vi "Datadashboard CD Main Page.vi"(8 "error in (no error)":errorcluster, 11 "Node Ptr":T1 format="%.0x") -> (0 "error out":errorcluster)   [LabVIEW 2013, in "Datadashboard CD Custom Device.lvlib"]
uses:
  Datadashboard CD Custom Device.lvlib
  <vilib>/NI Veristand/Custom Device API/Custom Device Item Ref.ctl
  <vilib>/Utility/miscctls.llb/LVRowAndColumnUnsignedTypeDef.ctl
  <vilib>/NI Veristand/Custom Device API/Get Item Property (Boolean).vi
  <vilib>/NI Veristand/Custom Device API/Get Item Property (String Array).vi
  <vilib>/NI Veristand/Custom Device API/Get Item Property (I32).vi
  <vilib>/NI Veristand/Custom Device API/Set Item Property (Variant).vi
  <vilib>/NI Veristand/Custom Device API/Set Item Property (String Array).vi
  <vilib>/NI Veristand/Custom Device API/Set Item Property (I32).vi
  <vilib>/NI Veristand/Custom Device API/Custom Device API.lvlib
  <vilib>/NI Veristand/Custom Device Tools/Custom Device Utility Library/Custom Device Utility Library.lvlib
  <vilib>/NI Veristand/Custom Device API/Custom Device Channel Type.ctl
  <vilib>/NI Veristand/Custom Device API/Custom Device Channel.ctl
panel:
  in  "Published Channels":i32[](listbox)
  in  "Decimation":i32=1 min=1
  in  "Remove":bool
  in  "Add Channels":bool
  in  "Header":cluster{"Section Name":string}={"Section Name"="Channel Group Settings"}
  in  "Description":string
  in  "Name":string
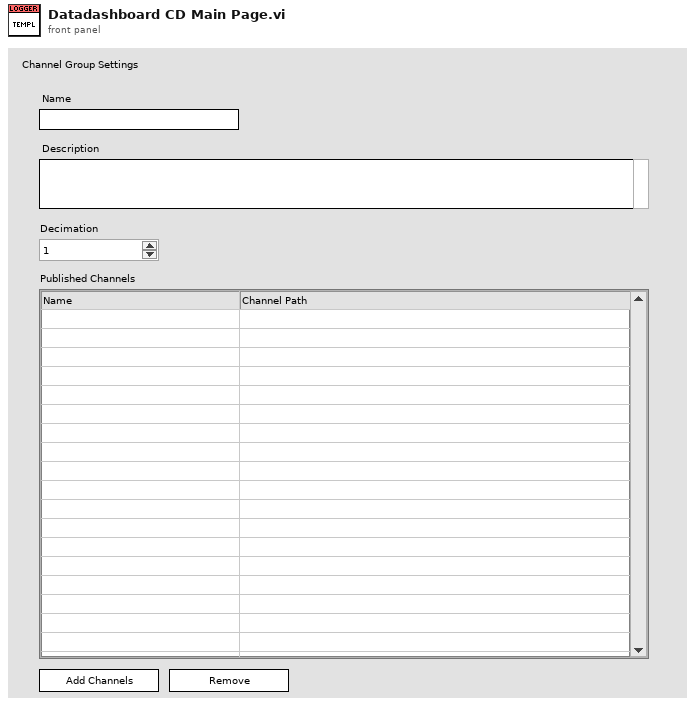
[diagram p1: front panel]
types:
  T1 = typedef "Custom Device API.lvlib/Custom Device Item Ref.ctl" = u64
  T2 = typedef "Custom Device API.lvlib/Custom Device Item Info.ctl" = cluster{"Name":string, "Is Channel":bool, "GUID":string, "Is Waveform":bool}
  T3 = typedef "LVRowAndColumnUnsignedTypeDef.ctl" = cluster{"Row":u32, "Column":u32}
  T4 = typedef "Custom Device API.lvlib/Custom Device Commands.ctl" = enum16{"Default", "Item renamed", "Shutdown", "Dynamic button pressed"}
  T5 = typedef "LVRowAndColumnTypeDef.ctl" = cluster{"Row":i32, "Column":i32}
  T6 = typedef "Custom Device API.lvlib/Custom Device Channel.ctl" = cluster{"Type":T7, "Units":string, "Default Value":dbl, "Faultable":bool, "Scalable":bool}
  T7 = typedef "Custom Device API.lvlib/Custom Device Channel Type.ctl" = enum16{"Input", "Output"}
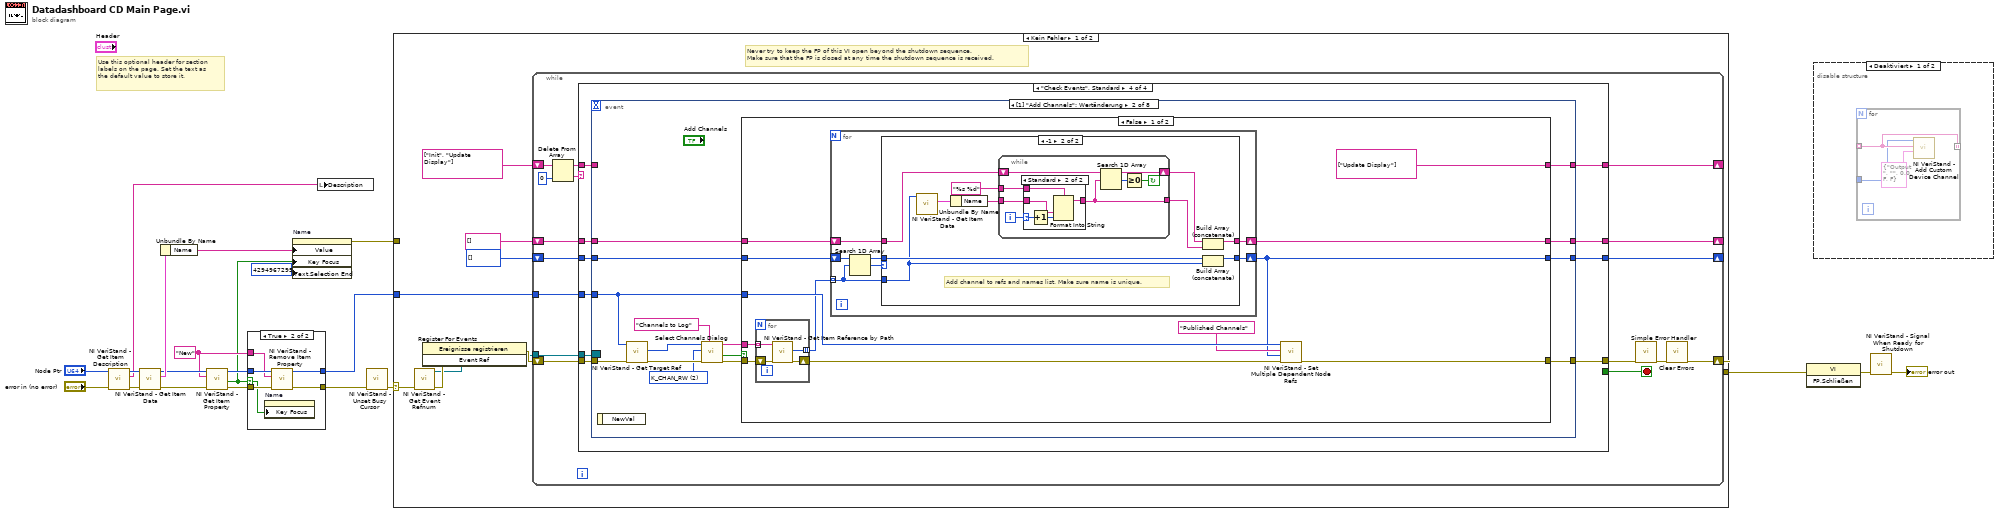
[diagram p0: block diagram]
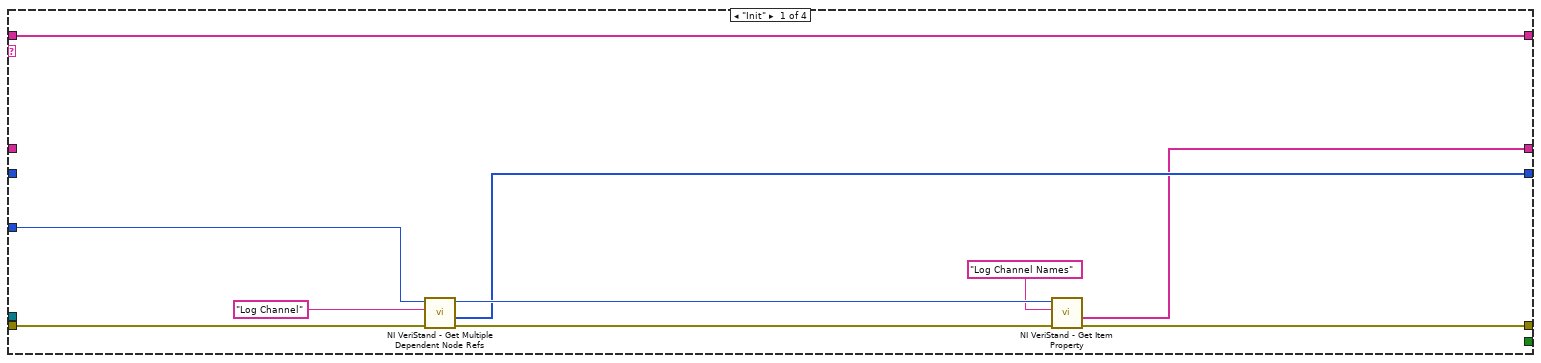
[diagram p4: hidden frame]
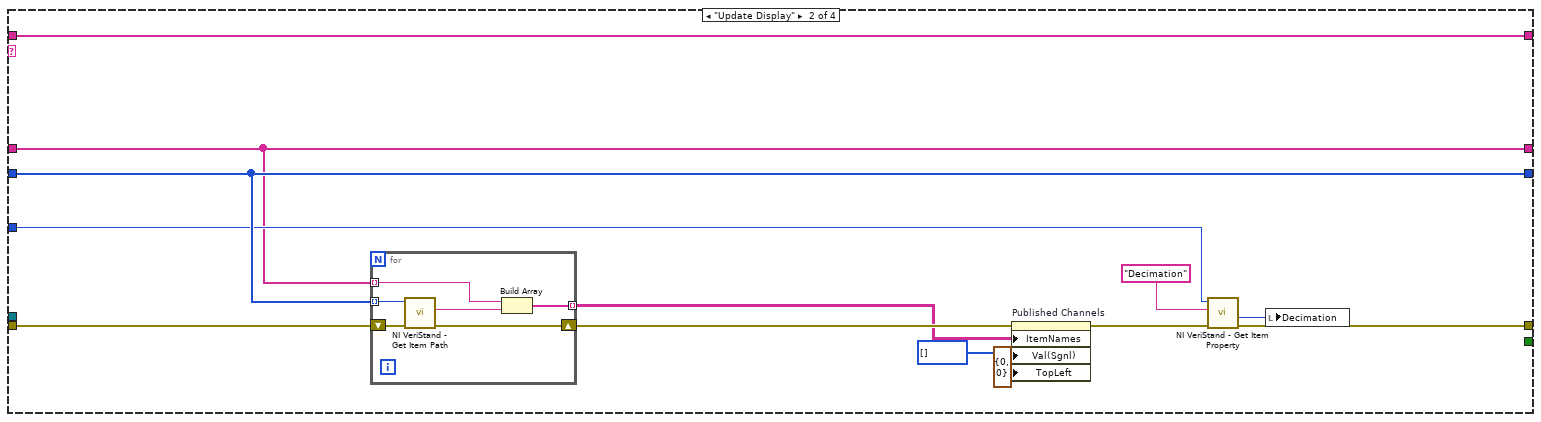
[diagram p5: hidden frame]
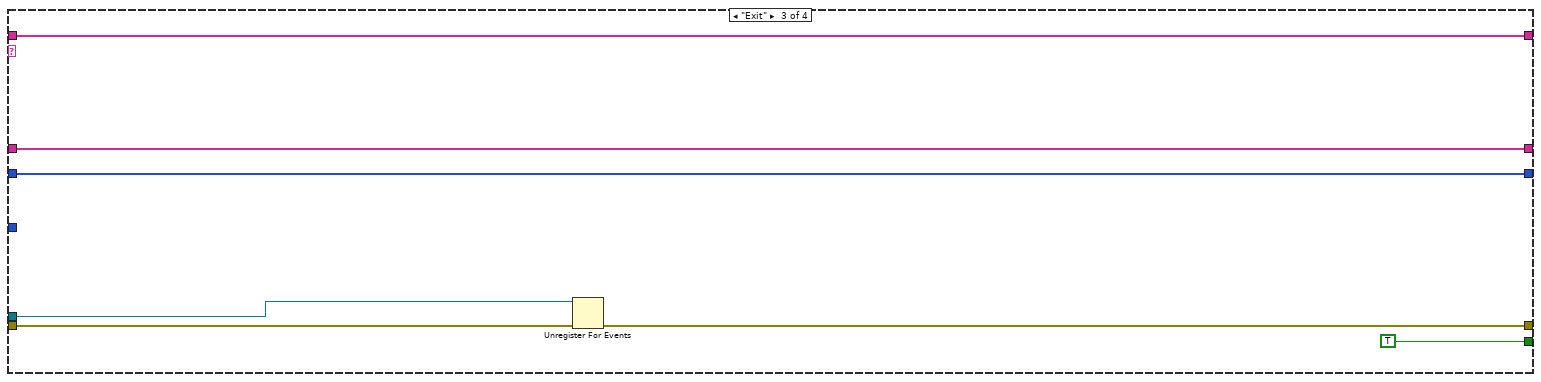
[diagram p6: hidden frame]
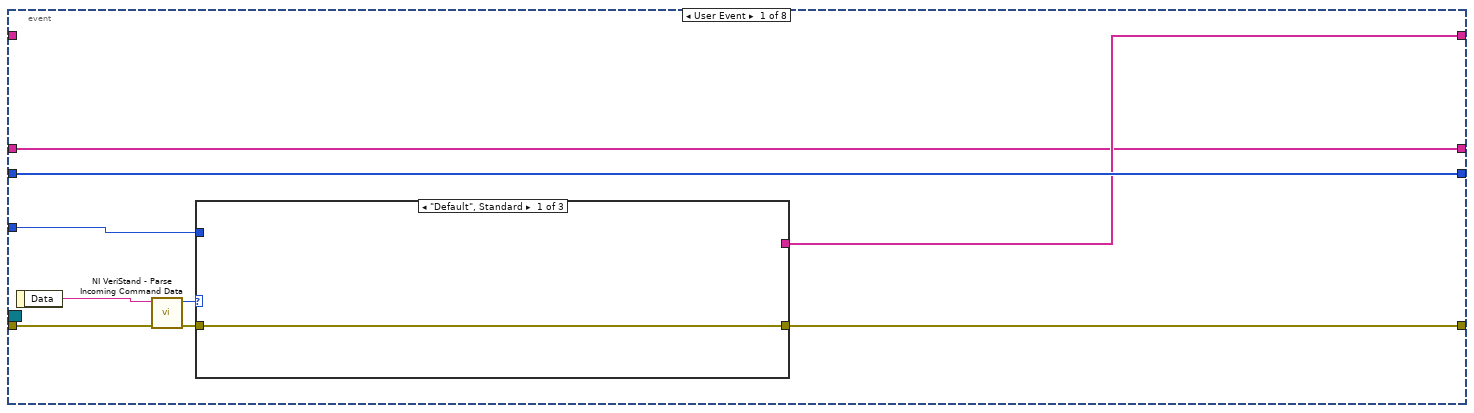
[diagram p7: hidden frame]
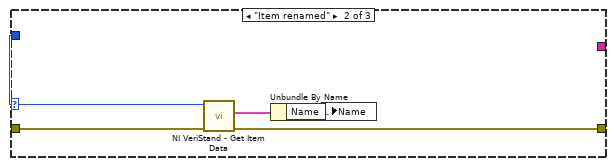
[diagram p8: hidden frame]
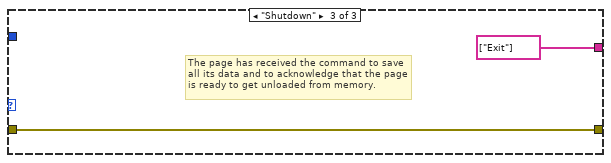
[diagram p9: hidden frame]
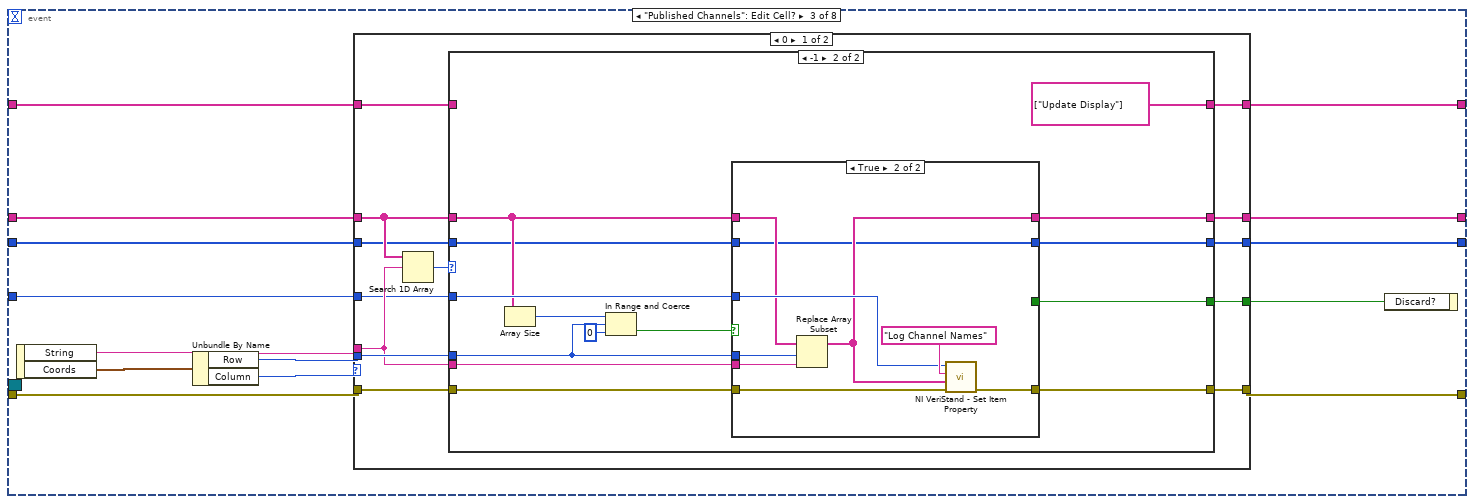
[diagram p13: hidden frame]
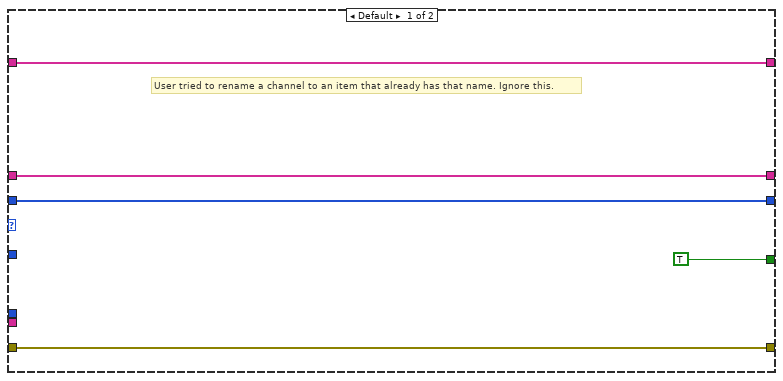
[diagram p14: hidden frame]
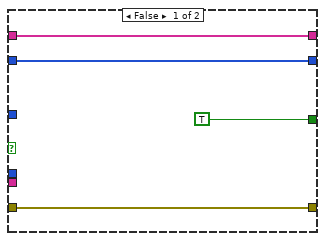
[diagram p15: hidden frame]
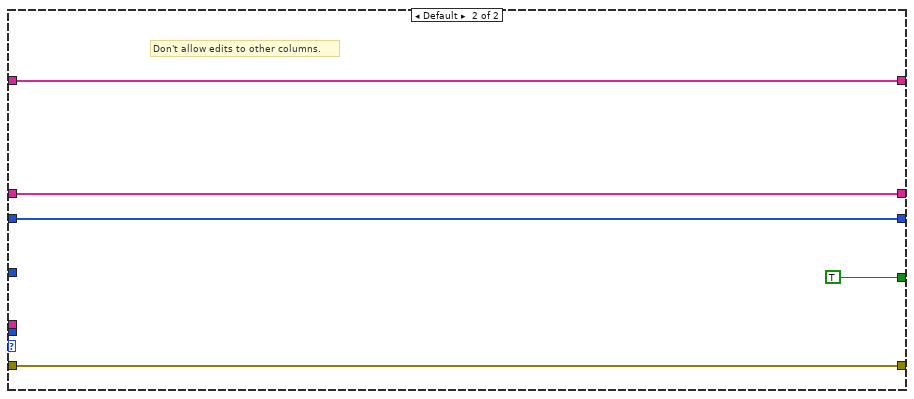
[diagram p16: hidden frame]
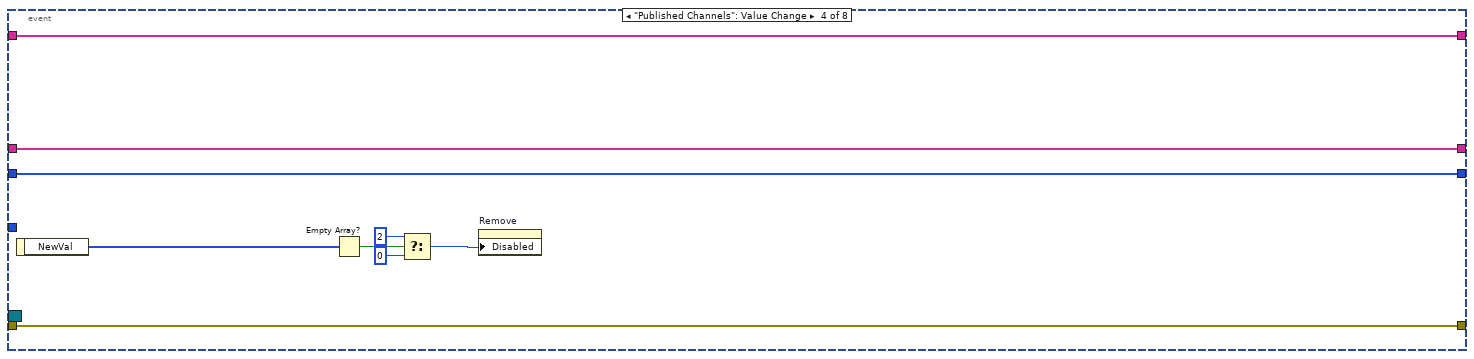
[diagram p17: hidden frame]
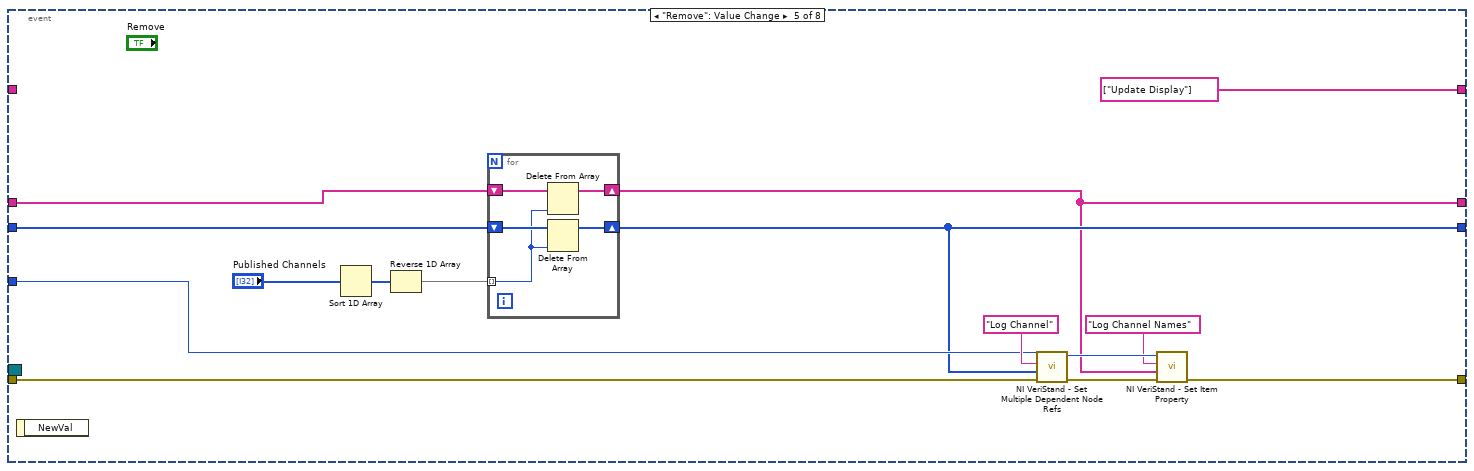
[diagram p18: hidden frame]
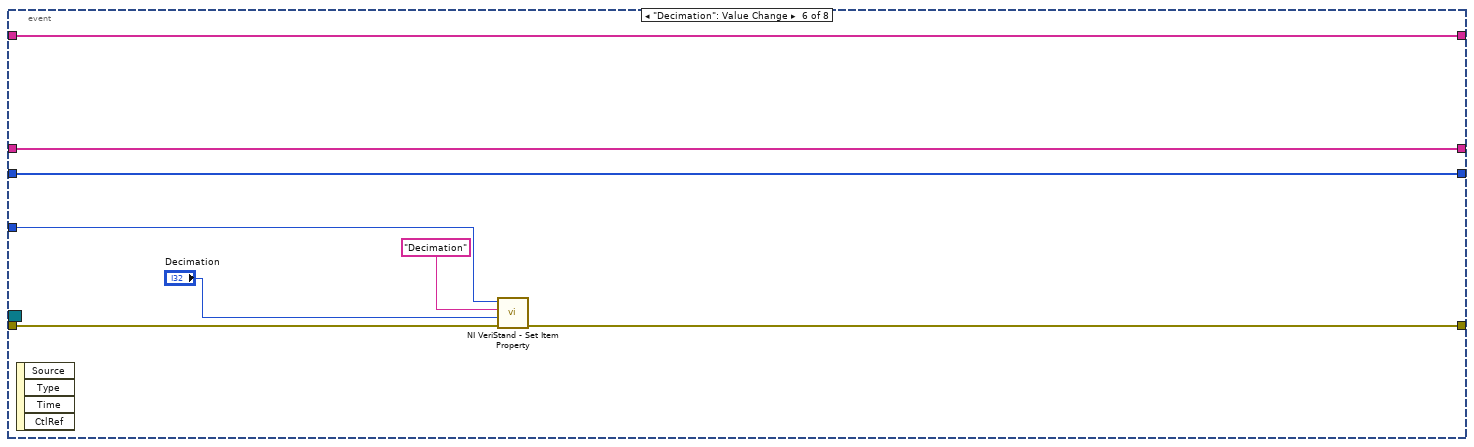
[diagram p19: hidden frame]
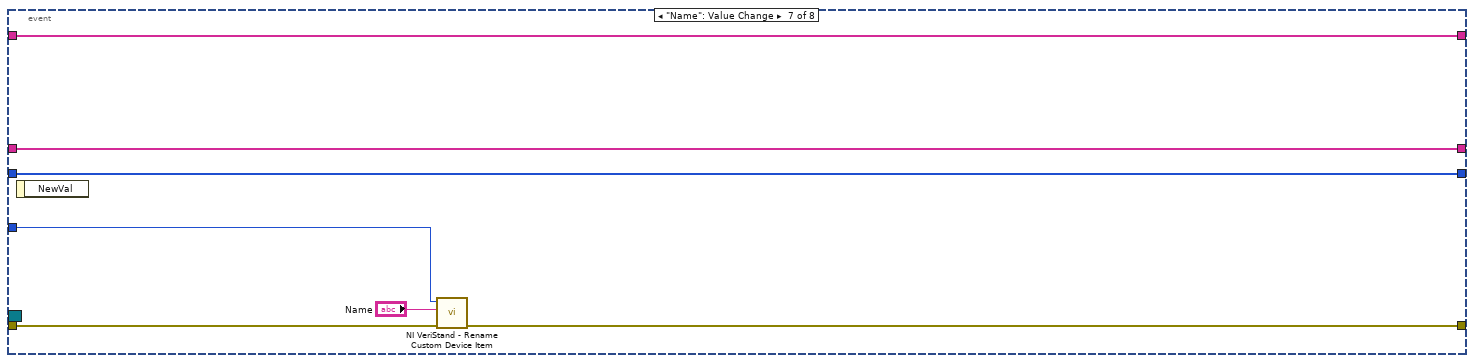
[diagram p20: hidden frame]
diagram:
  w6 = "New" ("Property Name")
  # "Use this optional header for section labels on the page. Set the text as the default value to store it."
  n1 = call <vilib>:"NI VeriStand - Get Item Description.vi"("error in (no error)"="error in (no error)", "Item Ref in"="Node Ptr") -> ("error out"=w14:errorcluster, "Description"=w15:string, "Item Ref out"=w16:T1)  [unwired: 7 out]
  n2 = call <vilib>:"NI VeriStand - Get Item Data.vi"("error in (no error)"=w14, "Item Ref in"=w16) -> ("error out"=w12:errorcluster, "Item Info"=w13:T2, "Item Ref out"=w11:T1)  [unwired: 7 out]
  n3 = Unbundle By Name(w13) -> ("Name"=w4:string)
  n4 = call-poly <vilib>:"NI VeriStand - Get Item Property.vi"("error in (no error)"=w12, "Property Name"=w6, "Item Ref in"=w11) -> ("error out"=w10:errorcluster, "Value"=w3:bool, "Item Ref out"=w8:T1)  [unwired: 5 in, 1 out]
  n5 = case shown="True" w3 {
    selector: w3 -> [_ w24]
    tunnel: w10 -> [w23 w28]
    tunnel: [w23 w25] -> w9
    tunnel: w8 -> [w22 w29]
    tunnel: [w22 w26] -> w7
    tunnel: w6 -> [_ w27]
    frame False {
    }
    frame True {
      n6 = property on="Name" class="Str"("Key Focus"=w24) -> ()  [unwired: 2 in, 2 out]
      n7 = call <vilib>:"NI VeriStand - Remove Item Property.vi"("error in (no error)"=w28, "Property Name"=w27, "Item Ref in"=w29) -> ("error out"=w25:errorcluster, "Item Ref out"=w26:T1)  [unwired: 6 in, 1 out]
    }
  }
  n8 = property on="Name" class="Str"("Value"=w4, "Key Focus"=w3, "Text.Selection End"=u32 4294967295 ("Text.Selection:End")) -> (error out=w2:errorcluster)  [unwired: 2 in, 1 out]
  n9 = local write "Description"(w15) -> ()
  n10 = call <vilib>:"NI VeriStand - Unset Busy Cursor.vi"("error in (no error)"=w9) -> ("error out"=w18:errorcluster)  [unwired: 10 out]
  n11 = case shown="Kein Fehler" w18 {
    selector: w18 -> [w34 w301]
    tunnel: [w31 w299] -> w21
    tunnel: w7 -> [w36 _]
    tunnel: w2 -> [_ _]
    frame No Error {
      # "Never try to keep the FP of this VI open beyond the shutdown sequence.\nMake sure that the FP is closed at any time the shutdown sequence is received."
      n12 = call <vilib>:"NI VeriStand - Get Event Refnum.vi"("error in (no error)"=w34) -> ("error out"=w39:errorcluster, "Event Ref"=w38:refnum<user-event>)  [unwired: 9 out]
      n13 = register-events(error in=w39, w38) -> (reference out=w32:refnum<event-registration>, error out=w37:errorcluster)  [unwired: 1 in]
      n14 = while {
        tunnel: w36 -> [w53]
        shift-right: [w50] -> w31
        shift-left: w37 -> [w55]
        shift-right: [w48] -> _
        shift-left: T1[] [] ("Selected Channel Refs") -> [w49]
        shift-right: [w44] -> _
        shift-left: string[] ["Init", "Update Display"] -> [w47]
        tunnel: w32 -> [w42]
        shift-right: [w40] -> _
        shift-left: string[] [] -> [w41]
        stop <- w54 stop-if-true
        n15 = Delete From Array(array=w47, index=0) -> (deleted portion=w43:string, array with subset deleted=w45:string[])  [unwired: 1 in]
        n16 = case shown="\"Check Events\", Standard" w43 {
          tunnel: w55 -> [w62 w78 w88 w101]
          tunnel: w42 -> [_ _ w86 w100]
          tunnel: [_ _ TRUE _] -> w54
          tunnel: w53 -> [w61 w74 _ w99]
          tunnel: [w56 w75 w87 w98] -> w52
          tunnel: w49 -> [_ w77 w91 w97]
          tunnel: [w59 w77 w91 w96] -> w48
          tunnel: w45 -> [w64 w70 w90 w95]
          tunnel: [w64 w70 w90 w94] -> w44
          tunnel: w41 -> [_ w66 w85 w93]
          tunnel: [w57 w66 w85 w92] -> w40
          frame "Init" {
            n17 = call <vilib>:"NI VeriStand - Get Multiple Dependent Node Refs.vi"("error in (no error)"=w62, "Base Property Name"="Log Channel", "Item Ref in"=w61) -> ("error out"=w58:errorcluster, "Dependent Node Refs"=w59:T1[], "Item Ref out"=w65:T1)  [unwired: 6 in]
            n18 = call-poly <vilib>:"NI VeriStand - Get Item Property.vi"("error in (no error)"=w58, "Property Name"="Log Channel Names", "Item Ref in"=w65) -> ("error out"=w56:errorcluster, "Value"=w57:string[])  [unwired: 1 in, 6 out]
          }
          frame "Update Display" {
            n19 = for {
              shift-right: [w82] -> w72
              shift-left: w78 -> [w84]
              tunnel: w77 -> [w83] mode=indexing
              tunnel: [w80] -> w71 mode=indexing
              tunnel: w66 -> [w79] mode=indexing
              n20 = call <vilib>:"NI VeriStand - Get Item Path.vi"("error in (no error)"=w84, "Item Ref in"=w83) -> ("error out"=w82:errorcluster, "Path"=w81:string)  [unwired: 8 out]
              n21 = Build Array(w79, w81) -> (w80:string[])
            }
            n22 = property on="Published Channels" class="MehrSpaltFeld (strikt)"(error in=w72, "ItemNames"=w71, "Val(Sgnl)"=i32[] [] ("Value (Signaling)"), "TopLeft"=T3 {"Row"=0, "Column"=0} ("Top Left Visible Cell")) -> (error out=w67:errorcluster)  [unwired: 1 in, 1 out]
            n23 = call-poly <vilib>:"NI VeriStand - Get Item Property.vi"("error in (no error)"=w67, "Property Name"="Decimation", "Item Ref in"=w74) -> ("error out"=w75:errorcluster, "Value"=w73:i32)  [unwired: 1 in, 6 out]
            n24 = local write "Decimation"(w73) -> ()
          }
          frame "Exit" {
            n25 = Unregister For Events(event registration refnum=w86, error in=w88) -> (error out=w87:errorcluster)
          }
          frame "Check Events", Default {
            n26 = event shown="[1] \"Add Channels\": Wertänderung" {
              selector: w100 -> [_ _ _ _ _ _ _ _]
              dyn-events: _ -> [_ _ _ _ _ _ _ _]
              timeout: _ -> [_ _ _ _ _ _ _ _]
              tunnel: w101 -> [w110 w123 w186 w250 w262 w282 w291 w297]
              tunnel: [w106 w128 w184 w250 w260 w278 w290 w296] -> w98
              tunnel: w99 -> [w105 w124 w185 _ w261 w280 w289 w298]
              tunnel: w97 -> [w104 w133 w196 w256 w270 w284 w287 w294]
              tunnel: [w104 w129 w193 w256 w258 w284 w287 w294] -> w96
              tunnel: w95 -> [_ _ w188 w255 _ w283 w286 w293]
              tunnel: [w103 w127 w187 w255 string[] ["Update Display"] w283 w286 w293] -> w94
              tunnel: w93 -> [w102 w126 w195 w248 w266 w277 w285 w292]
              tunnel: [w102 w125 w194 w248 w257 w277 w285 w292] -> w92
              event User Event {
                n27 = event-data() -> ("Data"=w109:string)  [unwired: 1 out]
                n28 = call <vilib>:"NI VeriStand - Parse Incoming Command Data.vi"("error in (no error)"=w110, "Incoming data"=w109) -> ("error out"=w108:errorcluster, "Action"=w107:T4)  [unwired: 8 out]
                n29 = case shown="\"Default\", Standard" w107 {
                  tunnel: w108 -> [w111 w116 w118]
                  tunnel: [w111 w113 w118] -> w106
                  tunnel: w105 -> [_ w115 _]
                  tunnel: [_ _ string[] ["Exit"]] -> w103
                  frame "Default", Default {
                  }
                  frame "Item renamed" {
                    n30 = call <vilib>:"NI VeriStand - Get Item Data.vi"("error in (no error)"=w116, "Item Ref in"=w115) -> ("error out"=w113:errorcluster, "Item Info"=w114:T2)  [unwired: 8 out]
                    n31 = Unbundle By Name(w114) -> ("Name"=w112:string)
                    n32 = local write "Name"(w112) -> ()
                  }
                  frame "Shutdown" {
                    # "The page has received the command to save all its data and to acknowledge that the page is ready to get unloaded from memory."
                  }
                }
              }
              event "Add Channels": Value Change {
                w119 = u8 2 items=["K_CHAN_R", "K_CHAN_W", "K_CHAN_RW", "K_CHAN_VOLT", "K_CHAN_FAULT", "K_ALL", "K_CUSTOM"] ("Filter")
                n33 = event-data() -> ()  [unwired: 2 out]
                n34 = call <vilib>:"NI VeriStand - Get Target Ref.vi"("error in"=w123, "Item Ref in"=w124) -> ("error out"=w122:errorcluster, "Target Ref"=w121:T1)  [unwired: 6 in, 2 out]
                n35 = call "Select Channels Dialog.vi"("Channel Label"="Channels to Log", "error in (no error)"=w122, "Filter"=w119, "Start Item Ref"=w121) -> ("error out"=w132:errorcluster, "Canceled"=w131:bool, "Channels"=w130:string[])  [unwired: 2 in, 3 out]
                n36 = case shown="False" w131 {
                  tunnel: w133 -> [w145 w183]
                  tunnel: w132 -> [w139 w182]
                  tunnel: w130 -> [w138 _]
                  tunnel: [w134 w183] -> w129
                  tunnel: [w140 w182] -> w128
                  tunnel: w124 -> [w142 _]
                  tunnel: [string[] ["Update Display"] _] -> w127
                  tunnel: w126 -> [w143 w181]
                  tunnel: [w135 w181] -> w125
                  frame False {
                    n37 = for {
                      shift-right: [w148] -> w136
                      shift-left: w139 -> [w149]
                      tunnel: w138 -> [w147] mode=indexing
                      tunnel: [w146] -> w137 mode=indexing
                      n38 = call <vilib>:"NI VeriStand - Get Item Reference by Path.vi"("error in (no error)"=w149, "Item Path in"=w147) -> ("error out"=w148:errorcluster, "Item Ref"=w146:T1)  [unwired: 6 in, 2 out]
                    }
                    n39 = for {
                      shift-right: [w153] -> w134
                      shift-left: w145 -> [w154]
                      shift-right: [w151] -> w135
                      shift-left: w143 -> [w152]
                      tunnel: w137 -> [w150] mode=indexing
                      n40 = Search 1D Array(1D array=w154, element=w150) -> (index of element=w155:i32)  [unwired: 1 out]
                      n41 = case shown="-1" w155 {
                        tunnel: w154 -> [w157 w167]
                        tunnel: [w157 w166] -> w153
                        tunnel: w150 -> [_ w165]
                        tunnel: w152 -> [w156 w160]
                        tunnel: [w156 w163] -> w151
                        frame Default {
                          # "Channel already selected for logging. Don't add to refs or names list."
                        }
                        frame -1 {
                          # "Add channel to refs and names list. Make sure name is unique."
                          n42 = call <vilib>:"NI VeriStand - Get Item Data.vi"("Item Ref in"=w165) -> ("Item Info"=w164:T2)  [unwired: 1 in, 9 out]
                          n43 = Unbundle By Name(w164) -> ("Name"=w159:string)
                          n44 = while {
                            shift-right: [w172] -> w161
                            shift-left: w160 -> [w172]
                            tunnel: w159 -> [w173]
                            tunnel: [w169] -> w158
                            tunnel: "%s %d" ("format string") -> [w168]
                            i -> [w174]
                            stop <- w170 continue-if-true
                            n45 = case shown="Standard" w174 {
                              selector: w174 -> [_ w178]
                              tunnel: w173 -> [w175 w176]
                              tunnel: [w175 w180] -> w169
                              tunnel: w168 -> [_ w179]
                              frame 0 {
                              }
                              frame Default {
                                n46 = Increment(x=w178) -> (x+1=w177:i32)
                                n47 = Format Into String(format string=w179, w176, w177) -> (resulting string=w180:string)  [unwired: 2 in, 1 out]
                              }
                            }
                            n48 = Search 1D Array(1D array=w172, element=w169) -> (index of element=w171:i32)  [unwired: 1 out]
                            n49 = Greater Or Equal To 0?(x=w171) -> (x >= 0?=w170:bool)
                          }
                          n50 = Build Array (concatenate)(w161, w158) -> (w163:string[])
                          n51 = Build Array (concatenate)(w167, w165) -> (w166:T1[])
                        }
                      }
                    }
                    n52 = call <vilib>:"NI VeriStand - Set Multiple Dependent Node Refs.vi"("error in (no error)"=w136, "Dependent Node Refs"=w134, "Base Property Name"="Published Channels" ("Property Name"), "Item Ref in"=w142) -> ("error out"=w140:errorcluster)  [unwired: 6 in, 1 out]
                  }
                  frame True {
                    # "User canceled out of the dialog."
                  }
                }
              }
              event "Published Channels": Edit Cell? {
                n53 = event-data() -> ("String"=w189:string, "Coords"=w197:T5)  [unwired: 1 out]
                n54 = Unbundle By Name(w197) -> ("Row"=w191:i32, "Column"=w192:i32)
                n55 = case shown="0" w192 {
                  tunnel: w196 -> [w203 w246]
                  tunnel: w195 -> [w205 w247]
                  tunnel: [w206 w247] -> w194
                  tunnel: [w204 w246] -> w193
                  tunnel: w191 -> [w202 _]
                  tunnel: [w209 TRUE] -> w190
                  tunnel: w189 -> [w201 _]
                  tunnel: w188 -> [w207 w244]
                  tunnel: [w208 w244] -> w187
                  tunnel: w186 -> [w200 w243]
                  tunnel: w185 -> [w199 _]
                  tunnel: [w198 w243] -> w184
                  frame 0 {
                    n56 = Search 1D Array(1D array=w205, element=w201) -> (index of element=w210:i32)  [unwired: 1 in]
                    n57 = case shown="-1" w210 {
                      tunnel: [TRUE w216] -> w209
                      tunnel: [w214 string[] ["Update Display"]] -> w208
                      tunnel: w207 -> [w214 _]
                      tunnel: [w213 w225] -> w206
                      tunnel: w205 -> [w213 w223]
                      tunnel: [w212 w222] -> w204
                      tunnel: w203 -> [w212 w221]
                      tunnel: w202 -> [_ w219]
                      tunnel: w201 -> [_ w228]
                      tunnel: w200 -> [w211 w227]
                      tunnel: w199 -> [_ w226]
                      tunnel: [w211 w224] -> w198
                      frame Default {
                        # "User tried to rename a channel to an item that already has that name. Ignore this."
                      }
                      frame -1 {
                        n58 = Array Size(array=w223) -> (size(s)=w220:i32)
                        n59 = In Range and Coerce(upper limit=w220, x=w219, lower limit=0) -> (In Range?=w218:bool)  [unwired: 1 out]
                        n60 = case shown="True" w218 {
                          tunnel: w219 -> [_ w242]
                          tunnel: w228 -> [_ w241]
                          tunnel: w227 -> [w231 w239]
                          tunnel: w226 -> [_ w238]
                          tunnel: [w233 w237] -> w225
                          tunnel: [w231 w236] -> w224
                          tunnel: w223 -> [w233 w235]
                          tunnel: [w232 w234] -> w222
                          tunnel: w221 -> [w232 w234]
                          tunnel: [TRUE _] -> w216
                          frame False {
                          }
                          frame True {
                            n61 = Replace Array Subset(array=w235, new element=w241, index=w242) -> (w237:string[])
                            n62 = call-poly <vilib>:"NI VeriStand - Set Item Property.vi"("error in (no error)"=w239, "Value"=w237, "Property Name"="Log Channel Names", "Item Ref in"=w238) -> ("error out"=w236:errorcluster)  [unwired: 7 out]
                          }
                        }
                      }
                    }
                  }
                  frame Default {
                    # "Don't allow edits to other columns."
                  }
                }
                n63 = event-data("Discard?"=w190) -> ()  [unwired: 1 in, 1 out]
              }
              event "Published Channels": Value Change {
                n64 = event-data() -> ("NewVal"=w249:i32[])  [unwired: 1 out]
                n65 = Empty Array?(array=w249) -> (empty?=w254:bool)
                n66 = Select(t=u8 2, s=w254, f=u8 0) -> (s? t:f=w251:u8)
                n67 = property on="Remove" class="Bool."("Disabled"=w251) -> ()  [unwired: 2 in, 2 out]
              }
              event "Remove": Value Change {
                n68 = event-data() -> ()  [unwired: 2 out]
                n69 = Sort 1D Array(array="Published Channels") -> (sorted array=w271:i32[])
                n70 = Reverse 1D Array(array=w271) -> (reversed array=w269:i32[])
                n71 = for {
                  shift-right: [w275] -> w258
                  shift-left: w270 -> [w276]
                  tunnel: w269 -> [w272] mode=indexing
                  shift-right: [w273] -> w257
                  shift-left: w266 -> [w274]
                  n72 = Delete From Array(array=w274, index=w272) -> (array with subset deleted=w273:string[])  [unwired: 1 in, 1 out]
                  n73 = Delete From Array(array=w276, index=w272) -> (array with subset deleted=w275:T1[])  [unwired: 1 in, 1 out]
                }
                n74 = call <vilib>:"NI VeriStand - Set Multiple Dependent Node Refs.vi"("error in (no error)"=w262, "Dependent Node Refs"=w258, "Base Property Name"="Log Channel" ("Property Name"), "Item Ref in"=w261) -> ("error out"=w259:errorcluster, "Item Ref out"=w264:T1)  [unwired: 6 in]
                n75 = call-poly <vilib>:"NI VeriStand - Set Item Property.vi"("error in (no error)"=w259, "Value"=w257, "Property Name"="Log Channel Names", "Item Ref in"=w264) -> ("error out"=w260:errorcluster)  [unwired: 5 in, 2 out]
              }
              event "Decimation": Value Change {
                n76 = event-data() -> ()  [unwired: 5 out]
                n77 = call-poly <vilib>:"NI VeriStand - Set Item Property.vi"("error in (no error)"=w282, "Value"="Decimation", "Property Name"="Decimation", "Item Ref in"=w280) -> ("error out"=w278:errorcluster)  [unwired: 7 out]
              }
              event "Name": Value Change {
                n78 = event-data() -> ()  [unwired: 2 out]
                n79 = call <vilib>:"NI VeriStand - Rename Custom Device Item.vi"("error in (no error)"=w291, "New Name"="Name", "Item Ref in"=w289) -> ("error out"=w290:errorcluster)  [unwired: 1 in, 7 out]
              }
              event "Description": Value Change {
                n80 = event-data() -> ()  [unwired: 2 out]
                n81 = call <vilib>:"NI VeriStand - Set Item Description.vi"("error in (no error)"=w297, "Description"="Description", "Item Ref in"=w298) -> ("error out"=w296:errorcluster)  [unwired: 8 out]
              }
            }
          }
        }
        n82 = call <vilib>:"Simple Error Handler.vi"("error in (no error)"=w52) -> ("error out"=w51:errorcluster)  [unwired: 1 in, 7 out]
        n83 = call <vilib>:"Clear Errors.vi"("error in (no error)"=w51) -> ("error out"=w50:errorcluster)  [unwired: 6 out]
      }
    }
    frame Error {
      n84 = call <vilib>:"Simple Error Handler.vi"("error in (no error)"=w301) -> ("error out"=w300:errorcluster)  [unwired: 1 in, 7 out]
      n85 = call <vilib>:"Clear Errors.vi"("error in (no error)"=w300) -> ("error out"=w299:errorcluster)  [unwired: 6 out]
    }
  }
  n86 = invoke class="VI" method="FP.Schließen"(error in=w21) -> (error out=w20:errorcluster)  [unwired: 2 in, 2 out]
  n87 = disable-structure shown="Deaktiviert" {
    frame Disabled {
      n88 = for {
        tunnel: _ -> [w303] mode=indexing
        tunnel: [w303] -> _ mode=indexing
        tunnel: _ -> [w302]
        n89 = call <vilib>:"NI VeriStand - Add Custom Device Channel.vi"("Channel"=T6 {"Type"=enum."Output", "Units"="", "Default Value"=0.0, "Faultable"=FALSE, "Scalable"=FALSE}, "Channel Name"=w303, "Parent Ref in"=w302) -> ()  [unwired: 5 in, 4 out]
      }
    }
    frame Enabled {
    }
  }
  n90 = call <vilib>:"NI VeriStand - Signal When Ready for Shutdown.vi"("error in (no error)"=w20) -> ("error out"=→"error out":errorcluster)  [unwired: 10 out]
